vi "Keys.vi"(8 "error in (no error)":errorcluster, 11 "Map in":refnum<class "ObjectMap.lvclass">) -> (0 "error out":errorcluster, 2 "Keys":string[](array[string]), 3 "Map out":refnum<class "ObjectMap.lvclass">)   [LabVIEW 2013, in "LapDog.Collections.v1.Maps.lvlib" / "ObjectMap.lvclass"]
doc: "Returns a copy of all keys in the map."
uses:
  ObjectMap.lvclass
  ObjectMap.lvclass/ObjectMap.ctl
  MapImp/MapImp.lvclass
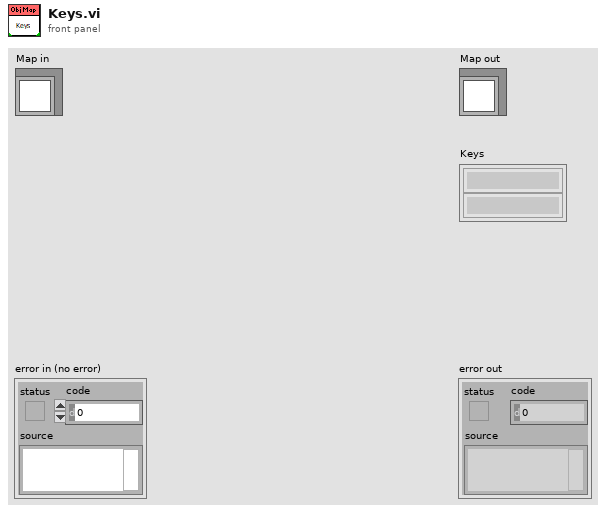
[diagram p1: front panel]
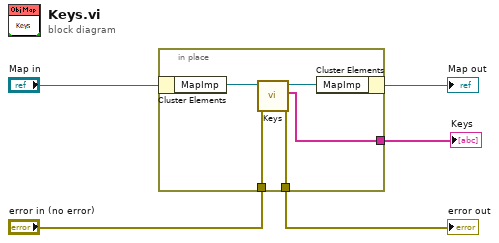
[diagram p0: block diagram]
diagram:
  n1 = in-place {
    in-place-border: "error in (no error)" -> [w8]
    in-place-border: [w7] -> w2
    in-place-border: [w6] -> w1
    n2 = in-place-cluster #1("Map in") -> ("MapImp"=w10:refnum<class "MapImp.lvclass">)
    n3 = call-dynamic "Keys.vi"("error in (no error)"=w8, "VariantAttribute in"=w10) -> ("error out"=w7:errorcluster, "Keys"=w6:string[], "VariantAttribute out"=w9:refnum<class "MapImp.lvclass">)  [unwired: 7 in]
    n4 = in-place-cluster #1("MapImp"=w9) -> (→"Map out":refnum<class "ObjectMap.lvclass">)
  }
  "error out" <- w2
  "Keys" <- w1
